vi "ComboBoz.vi"() -> ()   [LabVIEW 2019]
panel:
  out "String":string
  in  "Combo Box":string(combo)
  in  "Enum":T1(ring)
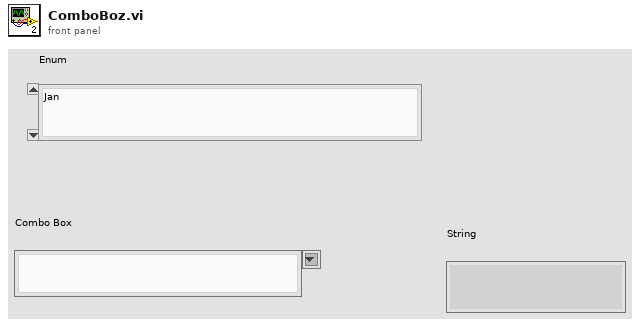
[diagram p1: front panel]
types:
  T1 = enum16{"Jan", "Feb", "Mar", "Apr", "May", "Jun", "jul", "Aug", "Sep", "Oct", "Nov", "Dec"}
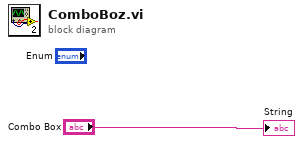
[diagram p0: block diagram]
diagram:
  "String" <- "Combo Box"
